vi "Sparse_Spd_Matrix.vi"(8 "error in (no error)":errorcluster caption="entrée d'erreur (pas d'erreur)", 11 "make_sparse_spd_matrix":T2={"dim"=1, "alpha"=0.95, "norm_diag"=FALSE, " smallest_coef"=0.1, "largest_coef"=0.9, "random_state"=-1} {"random_state" min=-1; "largest_coef" min=0.0 max=1.0; "smallest_coef" min=0.0 max=1.0; "alpha" min=0.0 max=1.0; "dim" min=1}) -> (0 "error out":errorcluster, 3 "Data":T1)   [LabVIEW 2020]
doc: "Generate a sparse symmetric definite positive matrix.\n\n\nParameters :\n\n- dim : integer, optional (default=1)\nThe size of the random matrix to generate.\n\n- alpha : float between 0 and 1, optional (default=0.95)\nThe probability that a coefficient is zero (see notes). Larger values enforce more sparsity.\n\n- norm_diag : boolean, optional (default=False)\nWhether to normalize the output matrix to make the leading diagonal elements all 1\n\n- smallest_coef : float between 0 and 1, optional (default=0.1)\nThe value of the smallest coefficient.\n\n- largest_coef : float between 0 and 1, optional (default=0.9)\nThe value of the largest coefficient.\n\n- random_state : int, RandomState instance, default=None=-1\nDetermines random number generation for dataset creation. Pass an int for reproducible output across multiple function calls. See Glossary.\n\nReturns : \n\n- prec : sparse matrix of shape (dim, dim)\nThe generated matrix."
uses:
  Sparse_Spd_Matrix.lvclass
panel:
  out "Sparse_Spd_Matrix.lvclass":refnum<class "Sparse_Spd_Matrix.lvclass">
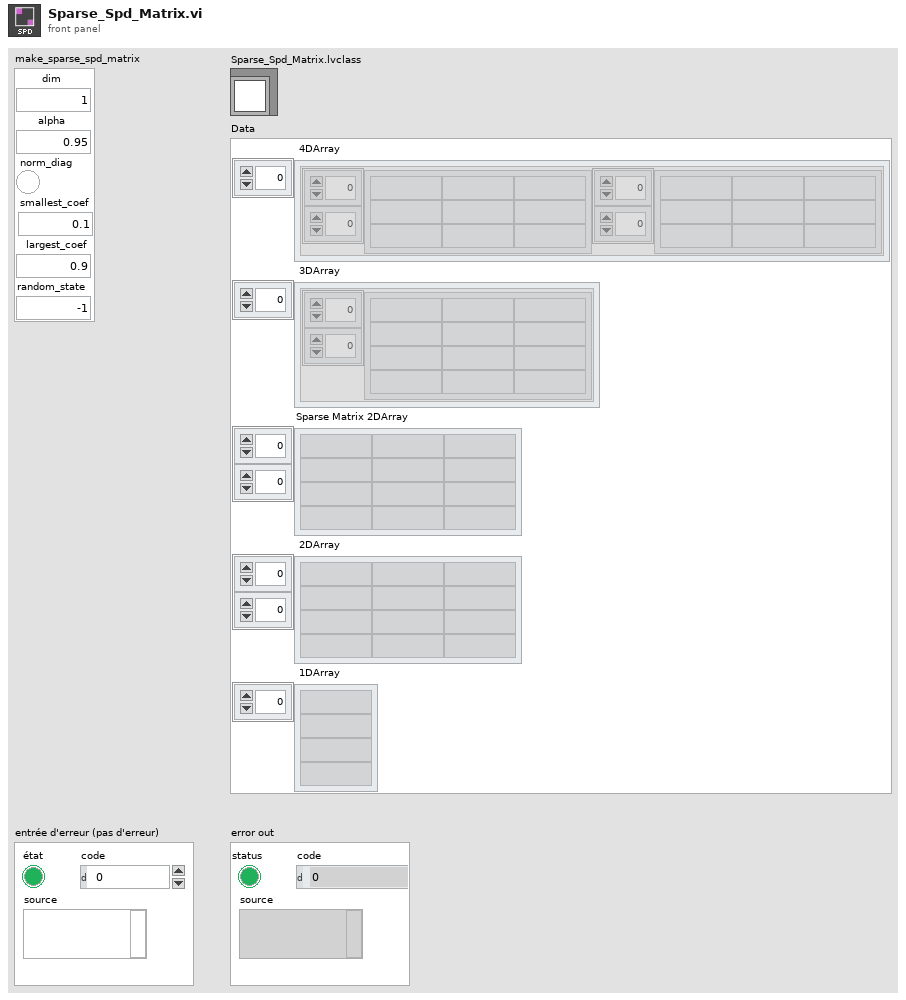
[diagram p1: front panel]
types:
  T1 = cluster{" 4DArray":cluster{"1":string[][], "2":string[][]}[], " 3DArray":cluster{"Tableau":string[][]}[], "Sparse Matrix 2DArray":string[][], " 2DArray":string[][], " 1DArray":string[]}
  T2 = cluster{"dim":u32, "alpha":dbl, "norm_diag":bool, " smallest_coef":dbl, "largest_coef":dbl, "random_state":i32}
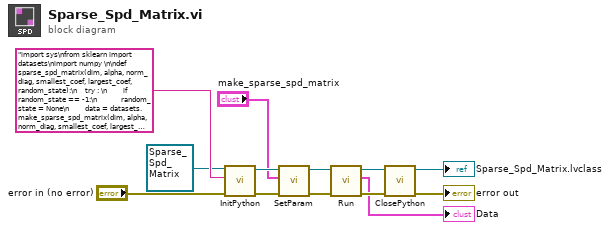
[diagram p0: block diagram]
diagram:
  n1 = call-dynamic "InitPython.vi"("error in (no error)"="error in (no error)", "Python Instruction"="import sys\nfrom sklearn import datasets\nimport numpy \n\ndef sparse_spd_matrix(dim, alpha, norm_diag, smallest_coef, largest_coef, random_state):\n    try : \n        if random_state == -1:\n            random_state = None\n        data = datasets.make_sparse_spd_matrix(dim, alpha, norm_diag, smallest_coef, largest_coef, random_state)\n        datas = data.tolist()\n        return str(datas)\n    except:\n        erreur = sys.exc_info()\n        typerr = u\"%s\" % (erreur[0])\n        typerr = typerr[typerr.find(\"'\")+1:typerr.rfind(\"'\")]\n        msgerr = u\"%s\" % (erreur[1])\n        message = str('/!\\\\ {0} : {1}'. format(typerr,msgerr))\n        return message", "Scikit-learn en entrée"=refnum<class "Sparse_Spd_Matrix.lvclass"> refnum ("Sparse_Spd_Matrix.lvclass")) -> ("error out"=w9:errorcluster, "Scikit-learn en sortie"=w10:refnum<class "Sparse_Spd_Matrix.lvclass">)  [unwired: 7 in]
  n2 = call-dynamic "SetParam.vi"("error in (no error)"=w9, "make_sparse_spd_matrix"="make_sparse_spd_matrix", "Sparse_Spd_Matrix.lvclass"=w10) -> ("error out"=w6:errorcluster, "Sparse_Spd_Matrix.lvclass"=w7:refnum<class "Sparse_Spd_Matrix.lvclass">)  [unwired: 7 in]
  n3 = call-dynamic "Run.vi"("error in (no error)"=w6, "Sparse_Spd_Matrix.lvclass"=w7) -> ("error out"=w4:errorcluster, "Data"=→"Data":T1, "Sparse_Spd_Matrix.lvclass"=w5:refnum<class "Sparse_Spd_Matrix.lvclass">)  [unwired: 7 in]
  n4 = call-dynamic "ClosePython.vi"("error in (no error)"=w4, "Scikit-learn en entrée"=w5) -> ("error out"=→"error out":errorcluster, "Scikit-learn en sortie"=→"Sparse_Spd_Matrix.lvclass":refnum<class "Sparse_Spd_Matrix.lvclass">)  [unwired: 8 in]
